vi "Test Sonar Sensors.vi"() -> ()   [LabVIEW 2011]
uses:
  <vilib>/LabVIEW Interface for Arduino/LabVIEW Interface for Arduino.lvlib
panel:
  in  "Threshold":dbl=100.0
  out "Right":bool
  out "Left":bool
  out "Front Right (Pin 2)":cluster{u32, u32}(slide) scale=0.0..1000.0
  out "Front Center (Pin 1)":cluster{u32, u32}(slide) scale=0.0..1000.0
  out "Front Left (Pin 0)":cluster{u32, u32}(slide) scale=0.0..1000.0
  in  "millisecond multiple":u32=100
  in  "Median Filter Rank":i32=10
  out "Analog Port":dbl[](array[numeric])
  in  "End Program":bool
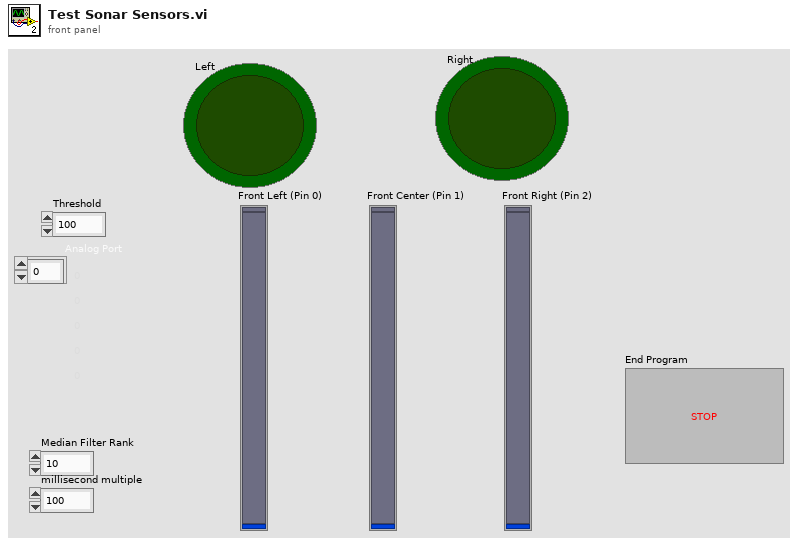
[diagram p1: front panel]
types:
  T1 = typedef "LabVIEW Interface for Arduino.lvlib/Arduino Resource.ctl" = cluster{"VISA resource":refnum<visa-resource-name>, "Board Type":T2, "Connection Type":enum8{"USB / Serial"}, "Bytes Per Packet (15)":u8}
  T2 = typedef "LabVIEW Interface for Arduino.lvlib/Board Type.ctl" = enum16{"Uno", "Dimuelanove w/Atmega 328", "Mega 2560"}
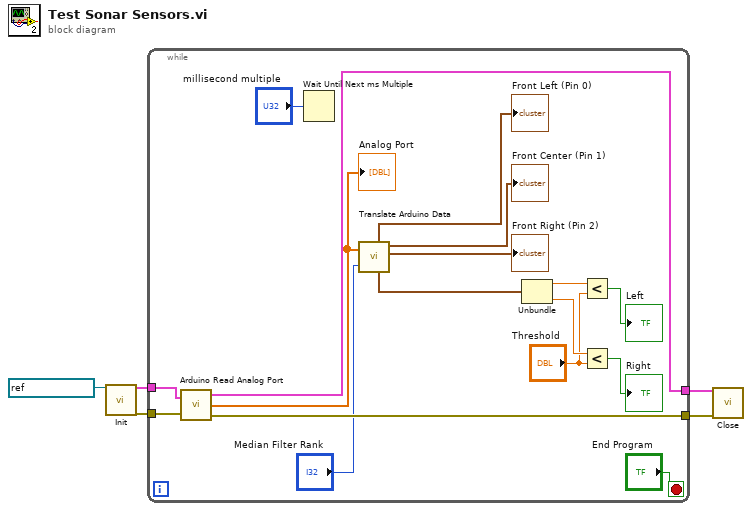
[diagram p0: block diagram]
diagram:
  n1 = call <vilib>:"Init.vi"("VISA resource"=refnum<visa-resource-name> "COM6") -> ("Arduino Resource"=w2:T1, "error out"=w1:errorcluster)  [unwired: 17 in]
  n2 = while {
    tunnel: w2 -> [w22]
    tunnel: w1 -> [w21]
    tunnel: [w20] -> w4
    tunnel: [w19] -> w3
    stop <- "End Program" stop-if-true
    n3 = call "Arduino Read Analog Port.vi"("Arduino Resource In"=w22, "Arduino Error In"=w21) -> ("Arduino Resource Out"=w20:T1, "Analog Port Out"=w16:dbl[], "Arduino Error Out"=w19:errorcluster)
    "Analog Port" <- w16
    n4 = Wait Until Next ms Multiple(millisecond multiple="millisecond multiple") -> ()  [unwired: 1 out]
    n5 = call "Translate Arduino Data.vi"("Analog Port In"=w16, "Median Filter Rank"="Median Filter Rank") -> ("Front Left (Pin 0)"=→"Front Left (Pin 0)":cluster{u32, u32}, "Sonar Data"=w11:cluster{dbl, dbl, dbl}, "Front Center (Pin 1)"=→"Front Center (Pin 1)":cluster{u32, u32}, "Front Right (Pin 2)"=→"Front Right (Pin 2)":cluster{u32, u32})  [unwired: 2 out]
    n6 = Unbundle(w11) -> (w9:dbl, w10:dbl)  [unwired: 1 out]
    n7 = Less?(x=w9, y="Threshold") -> (x < y?=→"Left":bool)
    n8 = Less?(x=w10, y="Threshold") -> (x < y?=→"Right":bool)
  }
  n9 = call <vilib>:"Close.vi"("Arduino Resource"=w4, "error in"=w3) -> ()  [unwired: 13 in, 1 out]
